vi "仁科设置说明.vi"() -> (3 "字符串":string)   [LabVIEW 2016, in "环境动力监测库.lvlib" / "空调库.lvlib"]
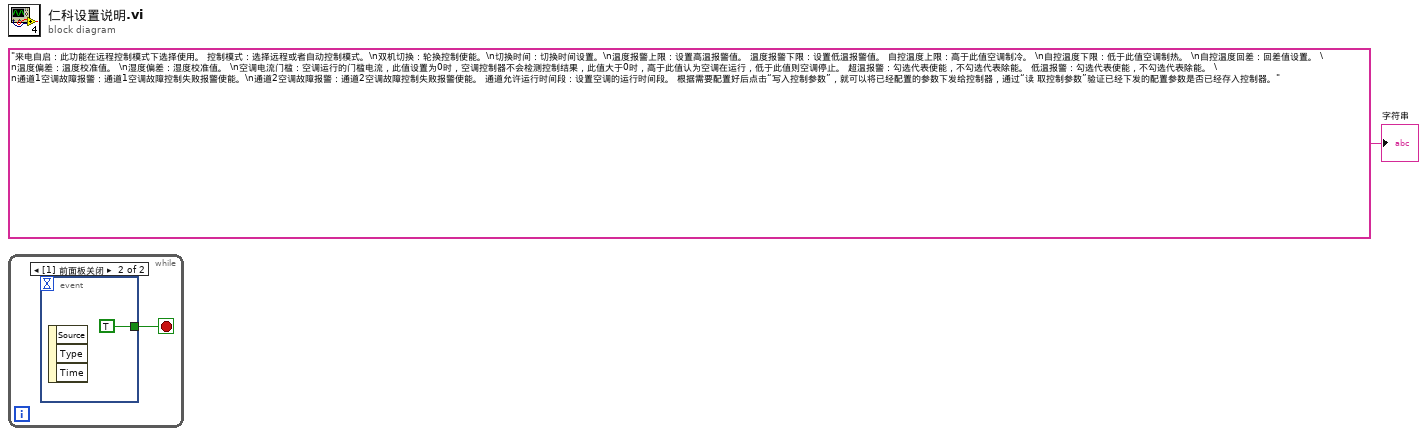
[diagram p0: block diagram]
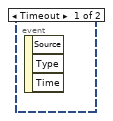
[diagram p2: hidden frame]
diagram:
  n1 = while {
    stop <- w2 stop-if-true
    n2 = event shown="[1] 前面板关闭" {
      selector: _ -> [_ _]
      dyn-events: _ -> [_ _]
      timeout: _ -> [_ _]
      tunnel: [_ TRUE] -> w2
      event Timeout {
        n3 = event-data() -> ()  [unwired: 1 in, 3 out]
      }
      event Panel Close {
        n4 = event-data() -> ()  [unwired: 1 in, 3 out]
      }
    }
  }
  "字符串" <- "来电自启：此功能在远程控制模式下选择使用。 控制模式：选择远程或者自动控制模式。\n双机切换：轮换控制使能。\n切换时间：切换时间设置。\n温度报警上限：设置高温报警值。 温度报警下限：设置低温报警值。 自控温度上限：高于此值空调制冷。 \n自控温度下限：低于此值空调制热。 \n自控温度回差：回差值设置。 \n温度偏差：温度校准值。 \n湿度偏差：湿度校准值。 \n空调电流门槛：空调运行的门槛电流，此值设置为0时，空调控制器不会检测控制结果，此值大于0时，高于此值认为空调在运行，低于此值则空调停止。 超温报警：勾选代表使能，不勾选代表除能。 低温报警：勾选代表使能，不勾选代表除能。 \n通道1空调故障报警：通道1空调故障控制失败报警使能。\n通道2空调故障报警：通道2空调故障控制失败报警使能。 通道允许运行时间段：设置空调的运行时间段。 根据需要配置好后点击“写入控制参数”，就可以将已经配置的参数下发给控制器，通过“读 取控制参数”验证已经下发的配置参数是否已经存入控制器。" ("字符串")
